vi "motor_test.vi"() -> ()   [LabVIEW 2019]
uses:
  <vilib>/addons/eal4LabVIEW/ApiLib/Connection control/ealApiConnect_string.vi
  <vilib>/addons/eal4LabVIEW/eal4LabVIEW.lvlib
panel:
  in  "stop":bool
  in  "condition":i32(ring) items=["AXIS_CONDITION_ACTIVE"=0, "AXIS_CONDITION_PARKING"=1, "AXIS_CONDITION_DEACTIVATED"=2, "AXIS_CONDITION_ACTIVE_DECOUPLED"=4, "AXIS_CONDITION_PARKING_DECOUPLED"=5, "AXIS_CONDITION_DEACTIVATED_DECOUPLED"=6, "AXIS_CONDITION_ACTIVE_PARAMETERIZATION"=8, "AXIS_CONDITION_PARKING_PARAMETERIZATION"=9, "AXIS_CONDITION_DEACTIVATED_PARAMETERIZATION"=10, "AXIS_CONDITION_ACTIVE_DECOUPLED_PARAMETERIZATION"=12, "AXIS_CONDITION_PARKING_DECOUPLED_PARAMETERIZATION"=13, "AXIS_CONDITION_DEACTIVATED_DECOUPLED_PARAMETERIZATION"=14]
  in  "slave index 6":i32
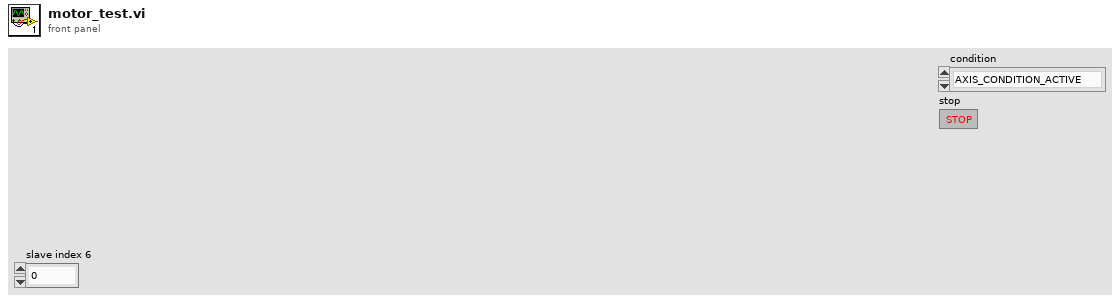
[diagram p1: front panel]
types:
  T1 = cluster{"Velocity":dbl, "Acceleration":dbl, "Deceleration":dbl, "Jerk":dbl}
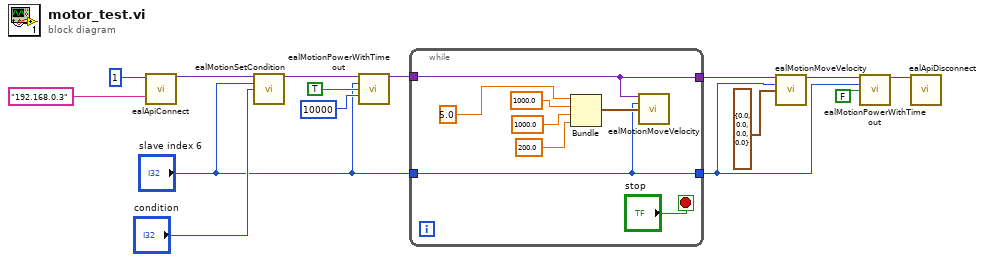
[diagram p0: block diagram]
diagram:
  n1 = call-poly <vilib>:"ealApiConnect.vi"("maximum no of axes"=1, "ip address"="192.168.0.3") -> ("connection out"=w9:variant)  [unwired: 12 in, 1 out]
  n2 = call <vilib>:"ealMotionSetCondition.vi"("connection in"=w9, "slave index"="slave index 6", "condition"="condition") -> ("connection out"=w8:variant)  [unwired: 11 in, 1 out]
  n3 = call <vilib>:"ealMotionPowerWithTimeout.vi"("connection in"=w8, "slave index"="slave index 6", "value"=TRUE, "timeout"=10000) -> ("connection out"=w5:variant)  [unwired: 10 in, 1 out]
  n4 = while {
    tunnel: w5 -> [w20]
    tunnel: [w20] -> w4
    tunnel: "slave index 6" -> [w17]
    tunnel: [w17] -> w1
    stop <- "stop" stop-if-true
    n5 = Bundle(5.0, 1000.0, 1000.0, 200.0) -> (w18:cluster{dbl, dbl, dbl, dbl})  [unwired: 1 in]
    n6 = call <vilib>:"ealMotionMoveVelocity.vi"("connection in"=w20, "slave index"=w17, "parameters set"=w18) -> ()  [unwired: 11 in, 2 out]
  }
  n7 = call <vilib>:"ealMotionMoveVelocity.vi"("connection in"=w4, "slave index"=w1, "parameters set"=T1 {"Velocity"=0.0, "Acceleration"=0.0, "Deceleration"=0.0, "Jerk"=0.0}) -> ("connection out"=w14:variant)  [unwired: 11 in, 1 out]
  n8 = call <vilib>:"ealMotionPowerWithTimeout.vi"("connection in"=w14, "slave index"=w1, "value"=FALSE) -> ("connection out"=w15:variant)  [unwired: 11 in, 1 out]
  n9 = call <vilib>:"ealApiDisconnect.vi"("connection in"=w15) -> ()  [unwired: 14 in, 1 out]
